vi "SaveImages.vi"(0 "object in":refnum<class "Experiment.lvclass">, 2 "Images":T1[](array[typedef]), 5 "error in (no error)":errorcluster) -> (14 "object out":refnum<class "Experiment.lvclass">, 16 "FileNames":string[](array[string]), 19 "error out":errorcluster)   [LabVIEW 2021, in "Experiment.lvclass"]
uses:
  Experiment.lvclass
  <vilib>/vision/Image Controls.llb/IMAQ Image.ctl
  Experiment.lvclass/Experiment.ctl
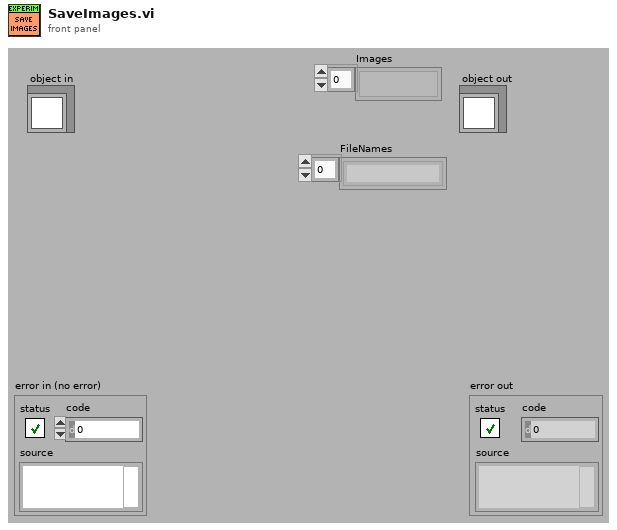
[diagram p1: front panel]
types:
  T1 = typedef "IMAQ Image.ctl" = refnum<image>
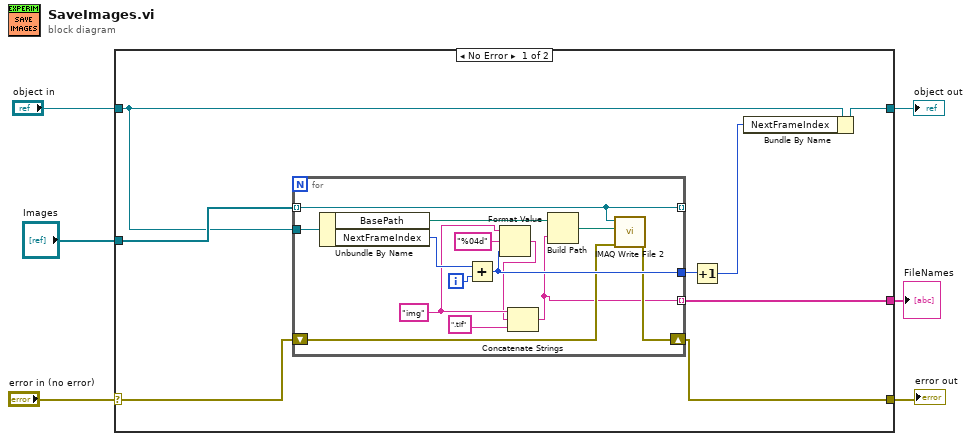
[diagram p0: block diagram]
diagram:
  n1 = case shown="No Error" "error in (no error)" {
    selector: "error in (no error)" -> [w9 w30]
    tunnel: [w8 w30] -> w5
    tunnel: [w11 w29] -> w3
    tunnel: "object in" -> [w13 w29]
    tunnel: "Images" -> [w14 _]
    tunnel: [w7 _] -> w1
    frame No Error {
      n2 = for {
        tunnel: w14 -> [w28] mode=indexing
        tunnel: [w28] -> _ mode=indexing
        tunnel: w13 -> [w27]
        tunnel: [w20] -> w12
        shift-right: [w18] -> w8
        shift-left: w9 -> [w19]
        tunnel: [w15] -> w7 mode=indexing
        i -> [w25]
        w21 = "img" ("string")
        n3 = Unbundle By Name(w27) -> ("BasePath"=w26:path, "NextFrameIndex"=w24:u16)
        n4 = Add(x=w24, y=w25) -> (x+y=w20:i32)
        n5 = Format Value(string ("")=w21, format string="%04d" ("format string (\" (%d)\")"), value (0)=w20) -> (output string=w16:string)
        n6 = Concatenate Strings(w21, w16, ".tif" ("string")) -> (w15:string)
        n7 = Build Path(base path=w26, name or relative path=w15) -> (appended path=w23:path)
        n8 = call-poly "IMAQ Write File 2"("error in (no error)"=w19, "File Path"=w23, "Image"=w28) -> ("error out"=w18:errorcluster)  [unwired: 7 in, 1 out]
      }
      n9 = Increment(x=w12) -> (x+1=w10:i32)
      n10 = Bundle By Name(cluster=w13, "NextFrameIndex"=w10) -> (w11:refnum<class "Experiment.lvclass">)
    }
    frame Error {
    }
  }
  "error out" <- w5
  "object out" <- w3
  "FileNames" <- w1
